vi "Wait for Stop.vi"(8 "error in (no error)":errorcluster, 10 "Timeout":i32=-1, 11 "bt_System in":refnum<class "bt_System.lvclass">) -> (0 "error":errorcluster, 1 "Status":T1, 2 "Timeout?":bool, 3 "bt_System out":refnum<class "bt_System.lvclass">)   [LabVIEW 2021, in "BT.lvlib" / "bt_System.lvclass"]
uses:
  bt_System.lvclass
  Support/Stop Status Type.ctl
  Support/Nodes/abs_Node/Status.ctl
  bt_System.lvclass/bt_System.ctl
  Support/Nodes/abs_Node/bt_Node.lvclass
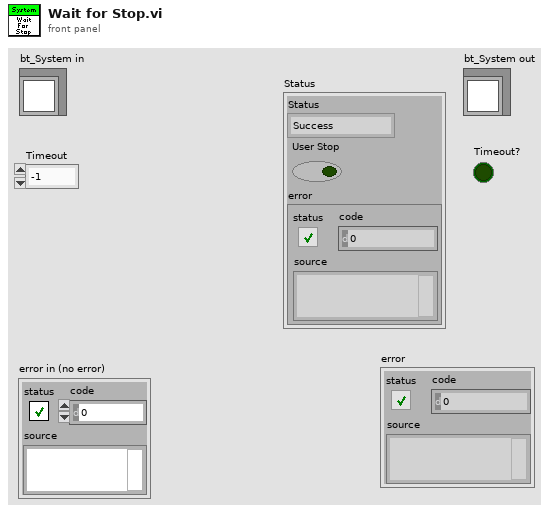
[diagram p1: front panel]
types:
  T1 = typedef "BT.lvlib/bt_System.lvclass/Stop Status Type.ctl" = cluster{"Status":T2, "User Stop":bool, "error":errorcluster}
  T2 = typedef "BT.lvlib/bt_Node.lvclass/Status.ctl" = enum16{"Success", "Failure", "Running"}
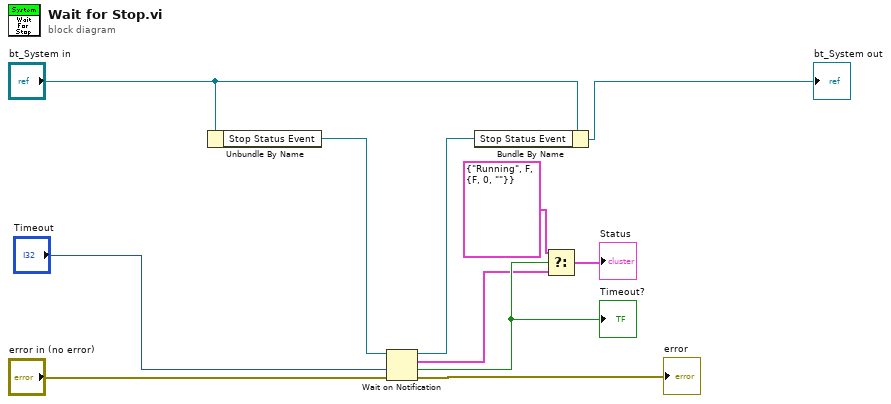
[diagram p0: block diagram]
diagram:
  n1 = Unbundle By Name("bt_System in") -> ("Stop Status Event"=w9:refnum<notifier>)
  n2 = Wait on Notification(notifier=w9, timeout in ms (-1)="Timeout", error in (no error)="error in (no error)") -> (notifier out=w8:refnum<notifier>, notification=w3:T1, timed out?=w4:bool, error out=→"error":errorcluster)  [unwired: 1 in]
  "Timeout?" <- w4
  n3 = Bundle By Name(cluster="bt_System in", "Stop Status Event"=w8) -> (→"bt_System out":refnum<class "bt_System.lvclass">)
  n4 = Select(t=T1 {"Status"=enum."Running", "User Stop"=FALSE, "error"={"status"=FALSE, "code"=0, "source"=""}}, s=w4, f=w3) -> (s? t:f=→"Status":T1)
